vi "WriteHeaders.vi"(0 "refnum in":refnum<file>, 5 "Match Number":u32, 7 "Date and Time":string, 9 "Battery Number":string, 11 "error in":errorcluster) -> (4 "refnum out":refnum<file>, 15 "error out":errorcluster)   [LabVIEW 2016]
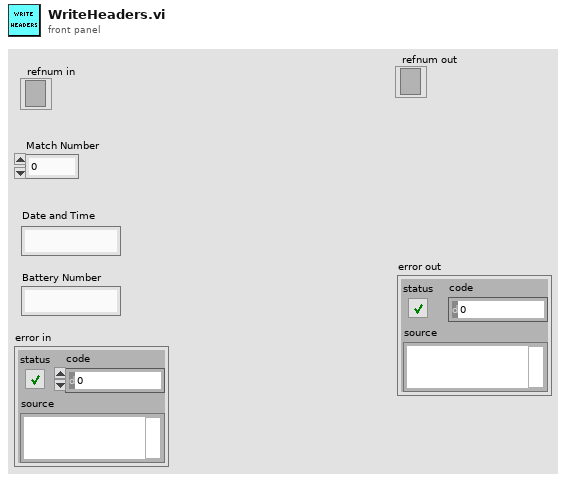
[diagram p1: front panel]
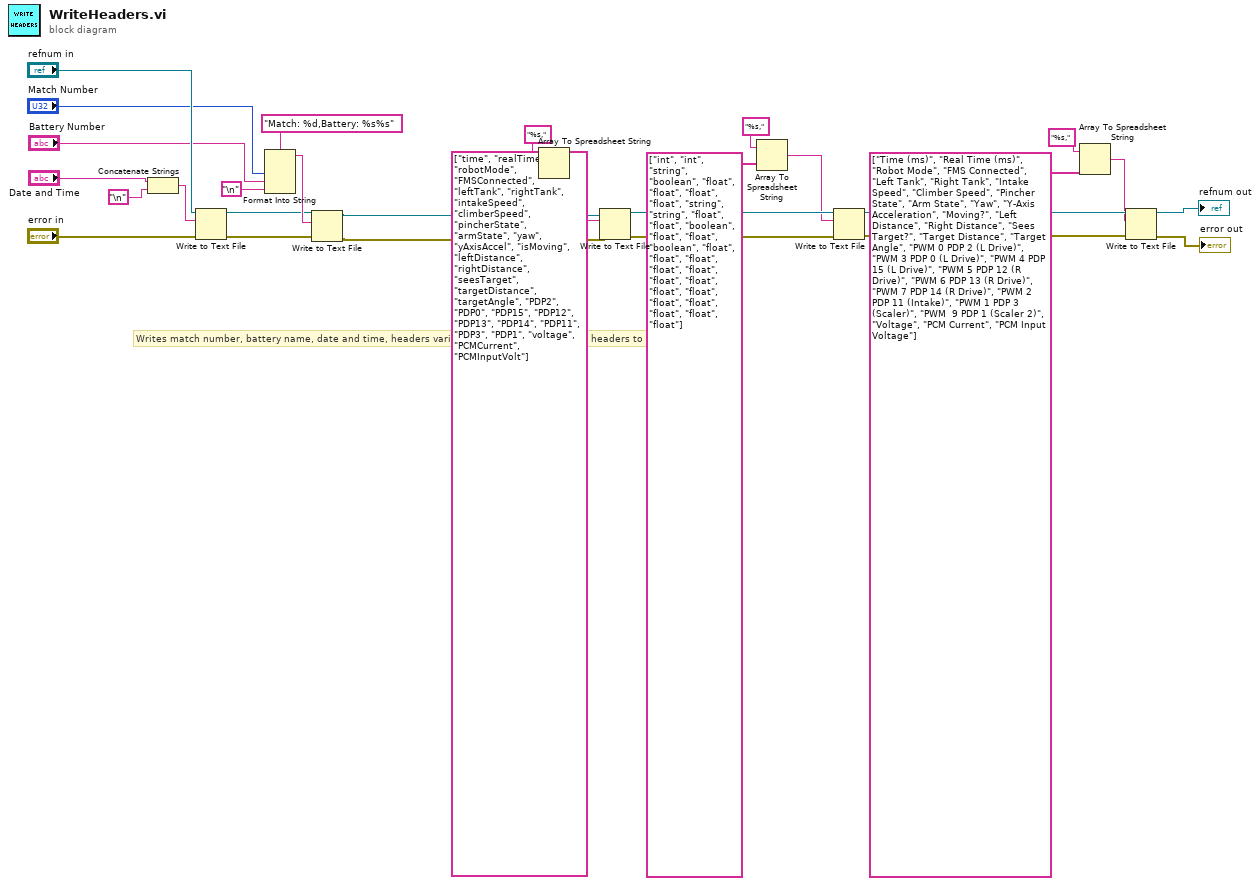
[diagram p0: block diagram]
diagram:
  # "Writes match number, battery name, date and time, headers variable names, data types, and headers to the log file"
  n1 = Concatenate Strings("Date and Time", "\n") -> (w27:string)
  n2 = Write to Text File(file (use dialog)="refnum in", text=w27, error in="error in") -> (refnum out=w21:refnum<file>, error out=w20:errorcluster)  [unwired: 1 in, 1 out]
  n3 = Format Into String(format string="Match: %d,Battery: %s%s", "Match Number", "Battery Number", "\n") -> (resulting string=w22:string)  [unwired: 2 in, 1 out]
  n4 = Write to Text File(file (use dialog)=w21, text=w22, error in=w20) -> (refnum out=w13:refnum<file>, error out=w12:errorcluster)  [unwired: 1 in, 1 out]
  n5 = Array To Spreadsheet String(array=string[] ["time", "realTime", "robotMode", "FMSConnected", "leftTank", "rightTank", "intakeSpeed", "climberSpeed", "pincherState", "armState", "yaw", "yAxisAccel", "isMoving", "leftDistance", "rightDistance", "seesTarget", "targetDistance", "targetAngle", "PDP2", "PDP0", "PDP15", "PDP12", "PDP13", "PDP14", "PDP11", "PDP3", "PDP1", "voltage", "PCMCurrent", "PCMInputVolt"], 3:"%s," ("format string")) -> (spreadsheet string=w5:string)  [unwired: 1 in]
  n6 = Write to Text File(file (use dialog)=w13, text=w5, error in=w12) -> (refnum out=w15:refnum<file>, error out=w14:errorcluster)  [unwired: 1 in, 1 out]
  n7 = Array To Spreadsheet String(array=string[] ["int", "int", "string", "boolean", "float", "float", "float", "float", "string", "string", "float", "float", "boolean", "float", "float", "boolean", "float", "float", "float", "float", "float", "float", "float", "float", "float", "float", "float", "float", "float", "float"], 3:"%s," ("format string")) -> (spreadsheet string=w4:string)  [unwired: 1 in]
  n8 = Write to Text File(file (use dialog)=w15, text=w4, error in=w14) -> (refnum out=w9:refnum<file>, error out=w8:errorcluster)  [unwired: 1 in, 1 out]
  n9 = Array To Spreadsheet String(array=string[] ["Time (ms)", "Real Time (ms)", "Robot Mode", "FMS Connected", "Left Tank", "Right Tank", "Intake Speed", "Climber Speed", "Pincher State", "Arm State", "Yaw", "Y-Axis Acceleration", "Moving?", "Left Distance", "Right Distance", "Sees Target?", "Target Distance", "Target Angle", "PWM 0 PDP 2 (L Drive)", "PWM 3 PDP 0 (L Drive)", "PWM 4 PDP 15 (L Drive)", "PWM 5 PDP 12 (R Drive)", "PWM 6 PDP 13 (R Drive)", "PWM 7 PDP 14 (R Drive)", "PWM 2 PDP 11 (Intake)", "PWM 1 PDP 3 (Scaler)", "PWM  9 PDP 1 (Scaler 2)", "Voltage", "PCM Current", "PCM Input Voltage"], 3:"%s," ("format string")) -> (spreadsheet string=w3:string)  [unwired: 1 in]
  n10 = Write to Text File(file (use dialog)=w9, text=w3, error in=w8) -> (refnum out=→"refnum out":refnum<file>, error out=→"error out":errorcluster)  [unwired: 1 in, 1 out]
